vi "Launch New Coms Instance.vi"(8 "Error In":errorcluster, 11 "Instance Details":T1) -> (0 "Error Out":errorcluster, 3 "Instance Details Out":T1)   [LabVIEW 2014]
uses:
  Controls/Known Aircraft.ctl
  Telemetry/Controls/Telemetry Connection Type.ctl
  Hardware Driver/Controls/Coms Driver Interface.ctl
  <vilib>/httpClient/ClientHandle.ctl
  <vilib>/httpClient/LabVIEWHTTPClient.lvlib
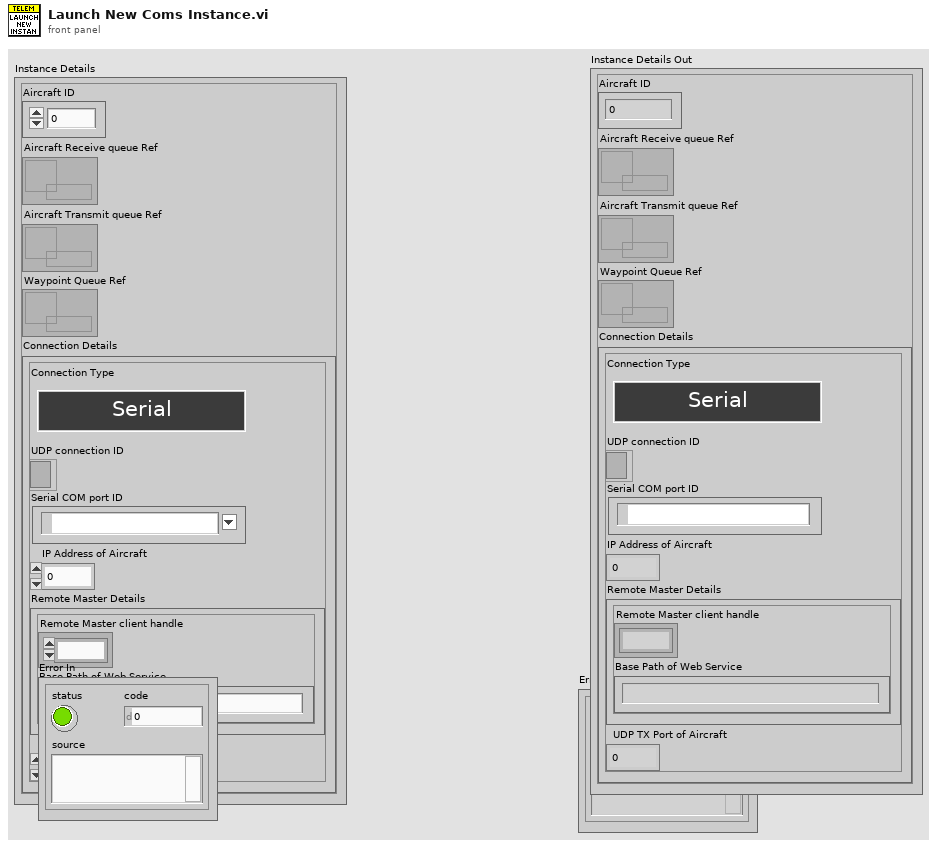
[diagram p1: front panel]
types:
  T1 = typedef "Known Aircraft.ctl" = cluster{"Aircraft ID":u8, "Aircraft Receive queue Ref":refnum<queue>, "Aircraft Transmit queue Ref":refnum<queue>, "Waypoint Queue Ref":refnum<queue>, "Connection Details":T2}
  T2 = typedef "Coms Driver Interface.ctl" = cluster{"Connection Type":T3, "UDP connection ID":refnum<k16>, "Serial COM port ID":refnum<visa-resource-name>, "IP Address of Aircraft":u32, "Remote Master Details":cluster{"Remote Master client handle":T4, "Base Path of Web Service":string}, "UDP TX Port of Aircraft":u16}
  T3 = typedef "Telemetry Connection Type.ctl" = enum16{"Serial", "UDP", "Remote Master"}
  T4 = typedef "LabVIEWHTTPClient.lvlib/ClientHandle.ctl" = refnum<k1>
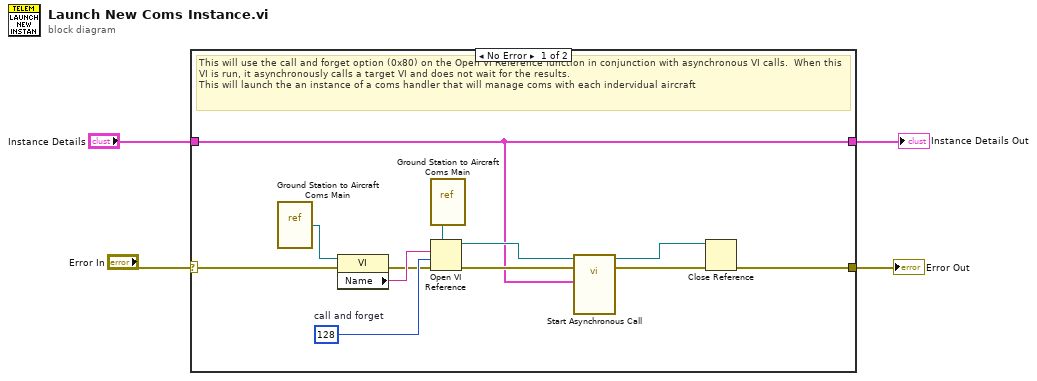
[diagram p0: block diagram]
diagram:
  n1 = case shown="No Error" "Error In" {
    selector: "Error In" -> [w7 w18]
    tunnel: [w8 w18] -> w4
    tunnel: "Instance Details" -> [w6 w17]
    tunnel: [w6 w17] -> w1
    frame No Error {
      w16 = 128  # call and forget
      # "This will use the call and forget option (0x80) on the Open VI Reference function in conjunction with asynchronous VI calls.  When this VI is run, it asynchronously calls a target VI and does not wait for the results.\nThis will launch the an instance of a coms handler that will manage coms with each indervidual aircraft"
      n2 = vi-ref "Ground Station to Aircraft Coms Main.vi"() -> (w11:refnum<vi>)
      n3 = property class="VI"(reference=w11, error in=w7) -> (error out=w9:errorcluster, "Name"=w10:string)  [unwired: 1 out]
      n4 = vi-ref "Ground Station to Aircraft Coms Main.vi"() -> (w5:refnum<vi>)
      n5 = Open VI Reference(type specifier VI Refnum (for type only)=w5, vi path=w10, options=w16, error in (no error)=w9) -> (vi reference=w15:refnum<vi>, error out=w14:errorcluster)  [unwired: 2 in]
      n6 = call-by-ref "Start Asynchronous Call"(reference=w15, error in=w14, "Instance Details"=w6) -> (reference out=w12:refnum<vi>, error out=w13:errorcluster)  [unwired: 11 in]
      n7 = Close Reference(reference=w12, error in (no error)=w13) -> (error out=w8:errorcluster)
    }
    frame Error {
    }
  }
  "Error Out" <- w4
  "Instance Details Out" <- w1
